vi "tearDown.vi"(8 "error in (no error)":errorcluster, 11 "reference in":refnum<class "TestCase.Pointer.lvclass">) -> (0 "error out":errorcluster, 3 "reference out":refnum<class "TestCase.Pointer.lvclass">)   [LabVIEW 2016, in "TestCase.Pointer.lvclass"]
doc: "tearDown runs after the test method has completed. Use this method to clean up any operations or references that were opened by setUp or the test method. Unit tests should be independent of other unit tests so this VI should ensure that the next test can run in a 'clean' test environment."
uses:
  TestCase.Pointer.lvclass
  TestCase.Pointer.lvclass/TestCase.Pointer.ctl
  Source/Classes/Internal/Memory.Pointer.Internal.lvclass
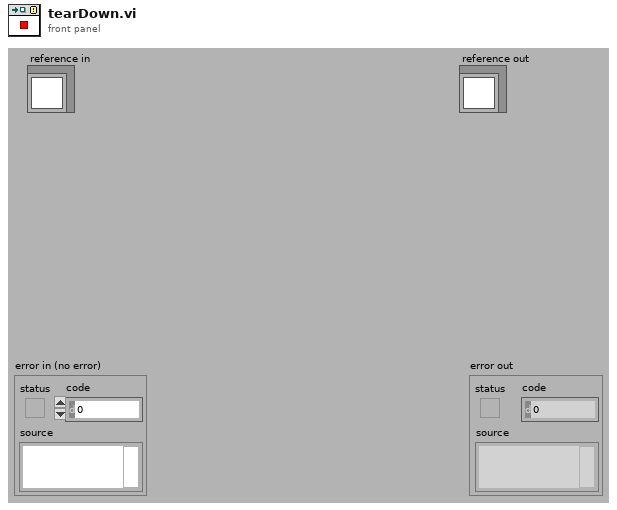
[diagram p1: front panel]
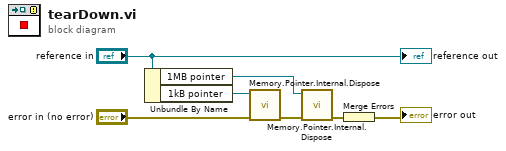
[diagram p0: block diagram]
diagram:
  n1 = Unbundle By Name("reference in") -> ("1MB pointer"=w1:refnum<class "Memory.Pointer.Internal.lvclass">, "1kB pointer"=w5:refnum<class "Memory.Pointer.Internal.lvclass">)
  n2 = call "Memory.Pointer.Internal.Dispose.vi"("error in (no error)"="error in (no error)", "pointer"=w5) -> ("error out"=w3:errorcluster)  [unwired: 9 in]
  n3 = call "Memory.Pointer.Internal.Dispose.vi"("error in (no error)"=w3, "pointer"=w1) -> ("error out"=w2:errorcluster)  [unwired: 9 in]
  n4 = Merge Errors(w2) -> (→"error out":errorcluster)
  "reference out" <- "reference in"
